vi "runServer.vi"(8 "error in (no error)":errorcluster, 11 "TcpServerCmd in":refnum<class "TcpServerCmd.lvclass">) -> (0 "error out":errorcluster, 3 "TcpServerCmd out":refnum<class "TcpServerCmd.lvclass">)   [LabVIEW 2018, in "TcpServerCmd.lvclass"]
doc: "Run the TCP Server Command.\n\nNOTE: Server Queue and Client Queue are destroyed in \"stop server\" state inside of tcpServerStateMachine.vi"
uses:
  TcpServerCmd.lvclass
  home/pcortes/github/ts_labview_tcp_json/src/TcpServerBase/TcpServerBase.lvclass
  TcpServerBase/typedef/tcpConnectionTypeDef.ctl
  TcpServerCmd.lvclass/TcpServerCmd.ctl
  TcpServerBase/TcpServerBase.lvclass/TcpServerBase.ctl
  typedef/eventTypeDef.ctl
  TcpServerBase/TcpServerBase.lvclass
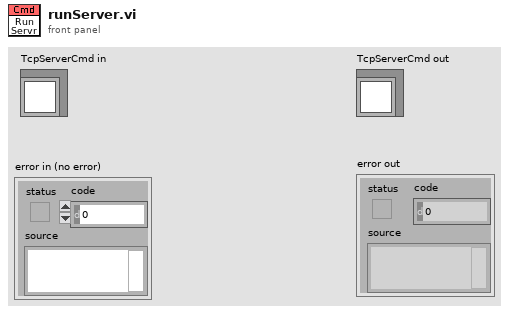
[diagram p1: front panel]
types:
  T1 = typedef "TcpServerBase.lvclass/tcpConnectionTypeDef.ctl" = cluster{"connection ID":refnum<k5>, "firstConnection":bool}
  T2 = typedef "TcpServerCmd.lvclass/userEventTypeDef.ctl" = cluster{"CmdRead":refnum<user-event>, "CmdWrite":refnum<user-event>, "EvtRead":refnum<user-event>, "EvtWrite":refnum<user-event>, "GenRead":refnum<user-event>, "GenWrite":refnum<user-event>}
  T3 = typedef "TcpServerCmd.lvclass/eventTypeDef.ctl" = cluster{"name":string, "evtlDetails":string}
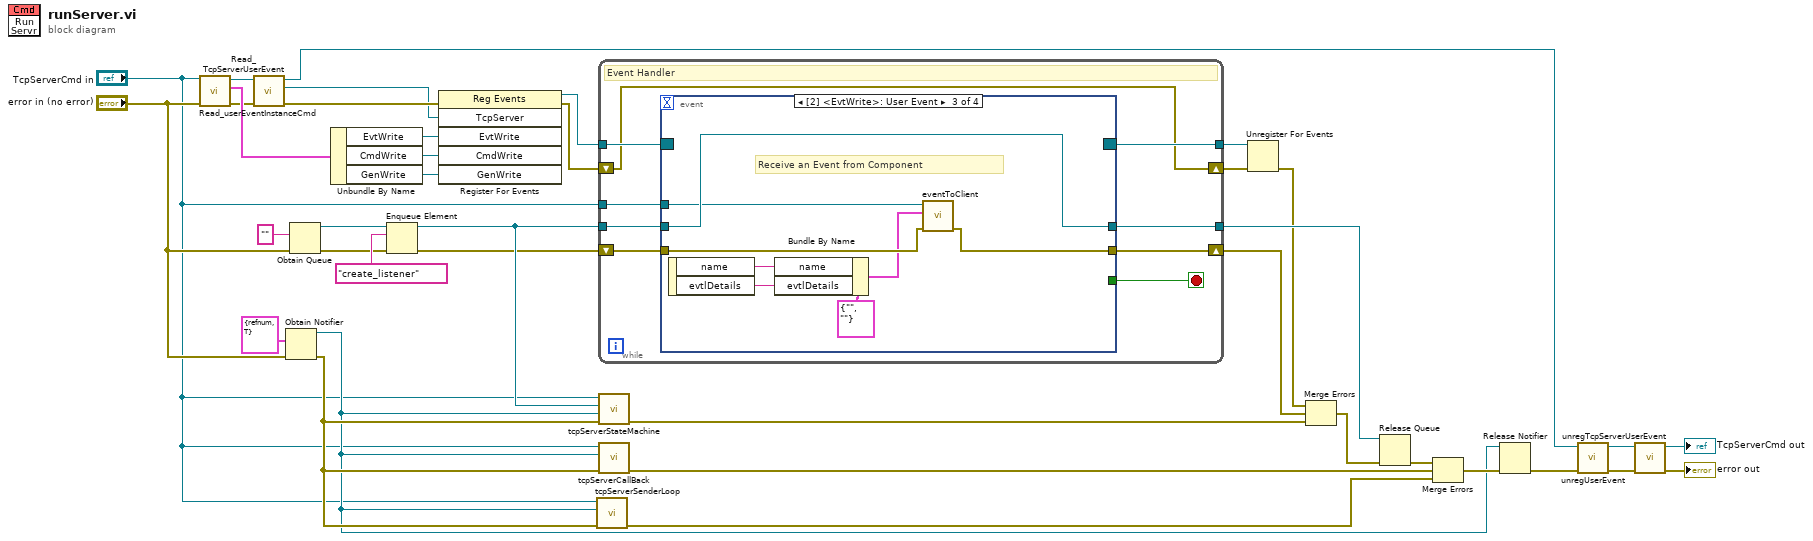
[diagram p0: block diagram]
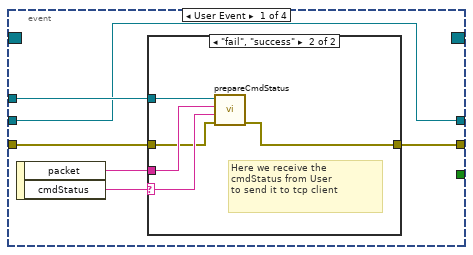
[diagram p2: hidden frame]
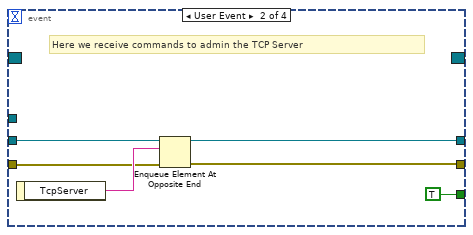
[diagram p4: hidden frame]
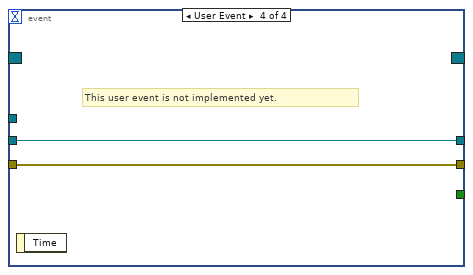
[diagram p5: hidden frame]
diagram:
  n1 = call "Read_userEventInstanceCmd.vi"("error in (no error)"="error in (no error)", "TcpServerCmd in"="TcpServerCmd in") -> ("error out"=w14:errorcluster, "userEventInstance"=w36:T2, "TcpServerCmd out"=w11:refnum<class "TcpServerCmd.lvclass">)  [unwired: 7 in]
  n2 = call "Read_TcpServerUserEvent.vi"("error in (no error)"=w14, "TcpServerBase in"=w11) -> ("error out"=w12:errorcluster, "TcpServer"=w10:refnum<user-event>, "TcpServerBase out"=w2:refnum<class "TcpServerCmd.lvclass">)  [unwired: 7 in]
  n3 = Obtain Notifier(notification data type=T1 {"connection ID"=refnum, "firstConnection"=TRUE} ("TcpConnectionCluster"), error in (no error)="error in (no error)") -> (notifier out=w4:refnum<notifier>, error out=w5:errorcluster)  [unwired: 2 in, 1 out]
  n4 = Obtain Queue(element data type="", error in (no error)="error in (no error)") -> (queue out=w37:refnum<queue>, error out=w26:errorcluster)  [unwired: 3 in, 1 out]
  n5 = Unbundle By Name(w36) -> ("EvtWrite"=w18:refnum<user-event>, "CmdWrite"=w29:refnum<user-event>, "GenWrite"=w15:refnum<user-event>)
  n6 = Enqueue Element(queue=w37, element="create_listener", error in (no error)=w26) -> (queue out=w34:refnum<queue>, error out=w24:errorcluster)  [unwired: 1 in, 1 out]
  n7 = register-events(error in=w12, w10, w18, w29, w15) -> (reference out=w35:refnum<event-registration>, error out=w23:errorcluster)  [unwired: 1 in]
  n8 = call "tcpServerSenderLoop.vi"("error in (no error)"=w5, "notifier in"=w4, "TcpServerBase in"="TcpServerCmd in") -> ("error out"=w27:errorcluster)  [unwired: 7 in, 1 out]
  n9 = while {
    tunnel: w34 -> [w47]
    tunnel: w35 -> [w46]
    tunnel: [w44] -> w32
    tunnel: "TcpServerCmd in" -> [w43]
    tunnel: [w42] -> w25
    shift-right: [w39] -> w21
    shift-left: w23 -> [w39]
    shift-right: [w40] -> w19
    shift-left: w24 -> [w41]
    stop <- w45 stop-if-true
    # "Event Handler"
    n10 = event shown="[2] <EvtWrite>: User Event" {
      selector: w46 -> [_ _ _ _]
      dyn-events: [_ _ _ _] -> w42
      timeout: _ -> [_ _ _ _]
      tunnel: w47 -> [w48 w65 w73 w74]
      tunnel: [_ TRUE _ _] -> w45
      tunnel: [w48 w62 w73 w74] -> w44
      tunnel: w43 -> [w51 _ w69 _]
      tunnel: w41 -> [w50 w61 w68 w75]
      tunnel: [w49 w60 w66 w75] -> w40
      event User Event {
        n11 = event-data() -> ("packet"=w52:string, "cmdStatus"=w53:string)  [unwired: 1 in]
        n12 = case shown="\"fail\", \"success\"" w53 {
          selector: w53 -> [_ w57]
          tunnel: w52 -> [_ w58]
          tunnel: w51 -> [_ w59]
          tunnel: w50 -> [w54 w56]
          tunnel: [w54 w55] -> w49
          frame Default {
          }
          frame "fail", "success" {
            # "Here we receive the \ncmdStatus from User \nto send it to tcp client"
            n13 = call "prepareCmdStatus.vi"("error in (no error)"=w56, "cmdStatus"=w57, "tcpPacket"=w58, "tcpServerCmd in"=w59) -> ("error out"=w55:errorcluster)  [unwired: 6 in, 1 out]
          }
        }
      }
      event User Event {
        # "Here we receive commands to admin the TCP Server"
        n14 = event-data() -> ("TcpServer"=w64:string)  [unwired: 1 in]
        n15 = Enqueue Element At Opposite End(queue=w65, element=w64, error in (no error)=w61) -> (queue out=w62:refnum<queue>, error out=w60:errorcluster)  [unwired: 1 in, 1 out]
      }
      event User Event {
        # "Receive an Event from Component"
        n16 = event-data() -> ("name"=w71:string, "evtlDetails"=w70:string)  [unwired: 1 in]
        n17 = Bundle By Name(cluster=T3 {"name"="", "evtlDetails"=""} ("eventConnID"), "name"=w71, "evtlDetails"=w70) -> (w67:T3)
        n18 = call "eventToClient.vi"("error in (no error)"=w68, "Event"=w67, "TcpServerCmd in"=w69) -> ("error out"=w66:errorcluster)  [unwired: 7 in, 1 out]
      }
      event User Event {
        # "This user event is not implemented yet."
        n19 = event-data() -> ()  [unwired: 1 in, 1 out]
      }
    }
  }
  n20 = call-dynamic "tcpServerStateMachine.vi"("error in (no error)"=w5, "notifier in"=w4, "tcpServerQueue"=w34, "TcpServerCmd in"="TcpServerCmd in") -> ("error out"=w31:errorcluster)  [unwired: 6 in, 1 out]
  n21 = call "tcpServerCallBack.vi"("error in (no error)"=w5, "notifier in"=w4, "TcpServerCmd in"="TcpServerCmd in") -> ("error out"=w28:errorcluster)  [unwired: 7 in, 1 out]
  n22 = Unregister For Events(event registration refnum=w25, error in=w21) -> (error out=w20:errorcluster)
  n23 = Merge Errors(w20, w19, w31) -> (w22:errorcluster)
  n24 = Release Queue(queue=w32, error in (no error)=w22) -> (error out=w30:errorcluster)  [unwired: 1 in, 2 out]
  n25 = Merge Errors(w30, w28, w27) -> (w17:errorcluster)
  n26 = Release Notifier(notifier=w4, error in (no error)=w17) -> (error out=w16:errorcluster)  [unwired: 1 in, 2 out]
  n27 = call "unregUserEvent.vi"("error in (no error)"=w16, "tcpServerCmd in"=w2) -> ("error out"=w8:errorcluster, "tcpServerCmd out"=w9:refnum<class "TcpServerCmd.lvclass">)  [unwired: 8 in]
  n28 = call "unregTcpServerUserEvent.vi"("error in (no error)"=w8, "tcpServerBase in"=w9) -> ("error out"=→"error out":errorcluster, "tcpServerBase out"=→"TcpServerCmd out":refnum<class "TcpServerCmd.lvclass">)  [unwired: 8 in]
